vi "Set separate code LVClass.vi"(8 "error in (no error)":errorcluster, 11 "File Path":path) -> (0 "error out":errorcluster, 1 "Saved":bool, 2 "Contains Compiled Code":bool)   [LabVIEW 2016]
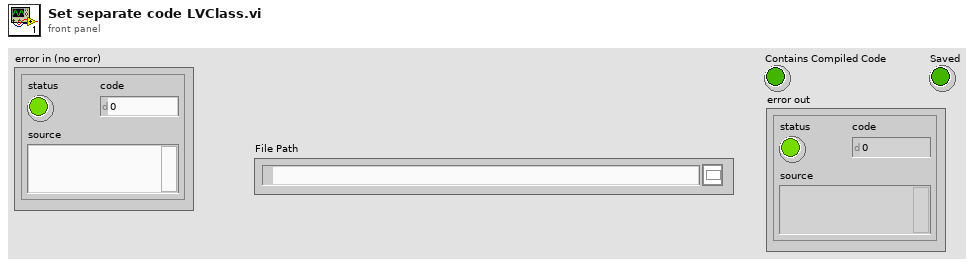
[diagram p1: front panel]
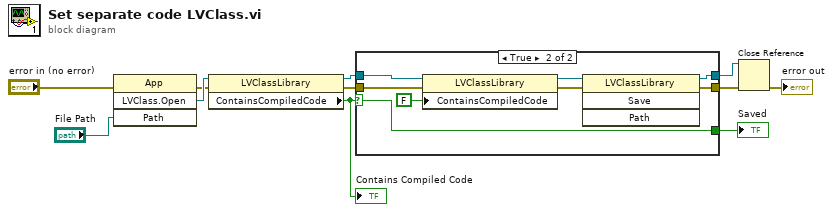
[diagram p0: block diagram]
diagram:
  n1 = invoke class="App" method="LVClass.Open"(error in="error in (no error)", "Path"="File Path") -> (error out=w9:errorcluster, "LVClass.Open"=w10:refnum<vi>)  [unwired: 2 in, 2 out]
  n2 = property class="LVClassLibrary"(reference=w10, error in=w9) -> (reference out=w7:refnum<vi>, error out=w6:errorcluster, "ContainsCompiledCode"=w8:bool)
  "Contains Compiled Code" <- w8
  n3 = case shown="True" w8 {
    selector: w8 -> [w12 w15]
    tunnel: w7 -> [w14 w22]
    tunnel: w6 -> [w13 w20]
    tunnel: [w13 w17] -> w4
    tunnel: [w14 w16] -> w5
    tunnel: [w12 w15] -> w1
    frame False {
    }
    frame True {
      n4 = property class="LVClassLibrary"(reference=w22, error in=w20, "ContainsCompiledCode"=FALSE ("Contains Compiled Code")) -> (reference out=w21:refnum<vi>, error out=w19:errorcluster)
      n5 = invoke class="LVClassLibrary" method="Save"(reference=w21, error in=w19) -> (reference out=w16:refnum<vi>, error out=w17:errorcluster)  [unwired: 2 in, 2 out]
    }
  }
  "Saved" <- w1
  n6 = Close Reference(reference=w5, error in (no error)=w4) -> (error out=→"error out":errorcluster)
